vi "Simulate Sine Signal.vi"(8 "error in (no error)":errorcluster) -> (0 "error out":errorcluster, 3 "Sine":dynamicdata(graph))   [LabVIEW 2023, in "Scope Simulated CFGs.lvlib" / "Fetch Waveforms CFG.lvclass"]
uses:
  Fetch Waveforms CFG.lvclass
  Fetch Waveforms CFG.lvclass/Fetch Waveforms CFG.ctl
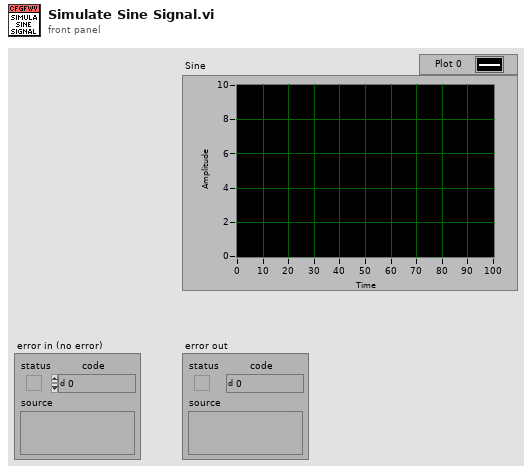
[diagram p1: front panel]
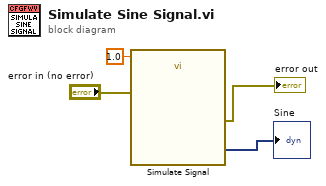
[diagram p0: block diagram]
diagram:
  n1 = call "Simulate Signal"("Offset"=1.0, "error in (no error)"="error in (no error)") -> ("Sine with Uniform Noise"=→"Sine":dynamicdata, "error out"=→"error out":errorcluster)  [unwired: 12 in]
